vi "atMonochromator_getEvent_DetailedState.vi"(8 "error in (no error)":errorcluster, 11 "logevent_DetailedState_Ctl":T1) -> (0 "error out":errorcluster, 2 "function return":i32, 3 "logevent_DetailedState_Ctl out":T1)   [LabVIEW 2016, in "SALLV_atMonochromator.lvlib"]
doc: "int atMonochromator_shm_getEvent_DetailedStateLV(atMonochromator_logevent_DetailedStateLV *logevent_DetailedState_Ctl );"
uses:
  SALLV_atMonochromator.lvlib
  DataTypes/logevent_DetailedState.ctl
  SALLV_atMonochromator.so
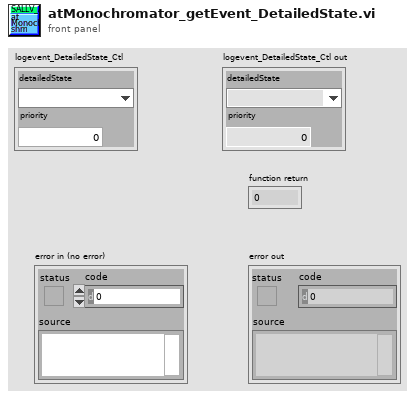
[diagram p1: front panel]
types:
  T1 = typedef "SALLV_atMonochromator.lvlib/logevent_DetailedState.ctl" = cluster{"detailedState":enum16{"", "DisabledState", "EnabledState", "FaultState", "OfflineState", "StandbyState", "MonoSettingUpState", "StoppedState", "StoppedCoolerOffState", "StoppedLightOffState", "StoppedLightOnState", "MonoManualSetup", "MonoAutomaticSetup"}, "priority":i32}
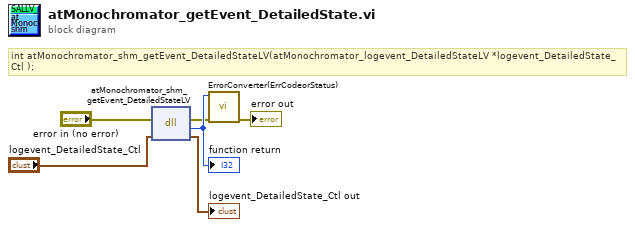
[diagram p0: block diagram]
diagram:
  # "int atMonochromator_shm_getEvent_DetailedStateLV(atMonochromator_logevent_DetailedStateLV *logevent_DetailedState_Ctl );"
  n1 = dll-call lib="home/andres/Desktop/SAL_atMonochromator/SALLV_atMonochromator.*" fn="atMonochromator_shm_getEvent_DetailedStateLV"(error in="error in (no error)", "logevent_DetailedState_Ctl"="logevent_DetailedState_Ctl") -> (error out=w2:errorcluster, w6:i32, "logevent_DetailedState_Ctl"=→"logevent_DetailedState_Ctl out":T1)  [unwired: 2 in, 1 out]
  "function return" <- w6
  n2 = call "ErrorConverter(ErrCodeorStatus).vi"("error in (no error)"=w2, "error code"=w6) -> ("error out"=→"error out":errorcluster)  [unwired: 9 in]
